vi "controlZLockIn.vi"(4 "thrAng":dbl=4.0 format="%#_13g", 6 "stop":bool, 7 "thr":dbl, 8 "error in (no error)":errorcluster, 9 "Tipo":enum16{"Amplitud", "Fase"}(ring), 10 "name":string, 11 "Distancia de medicion":dbl) -> (0 "error out":errorcluster, 1 "Act. Z":bool, 2 "limite":bool, 5 "Distancia Nano Z Act.":dbl)   [LabVIEW 2018]
uses:
  <vilib>/Utility/file.llb/Write Delimited Spreadsheet (DBL).vi
panel:
  out "Cerca":bool
  out "Fase":dbl[](graph)
  out "Thr":bool
  out "Amplitud":dbl[](graph)
  in  "stop 2":bool
  out "CambioZ":dbl
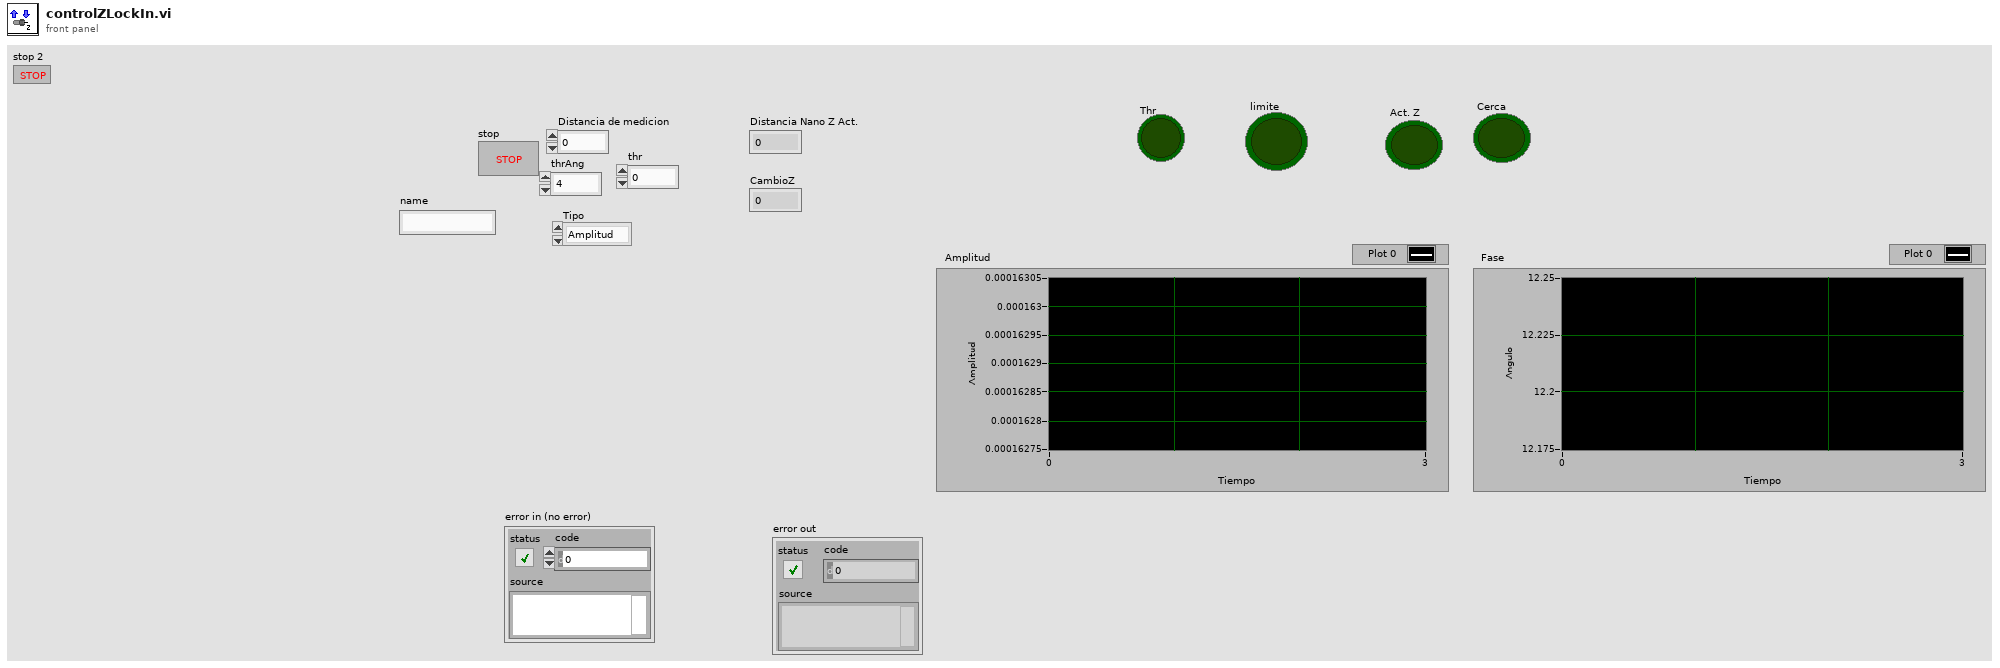
[diagram p1: front panel]
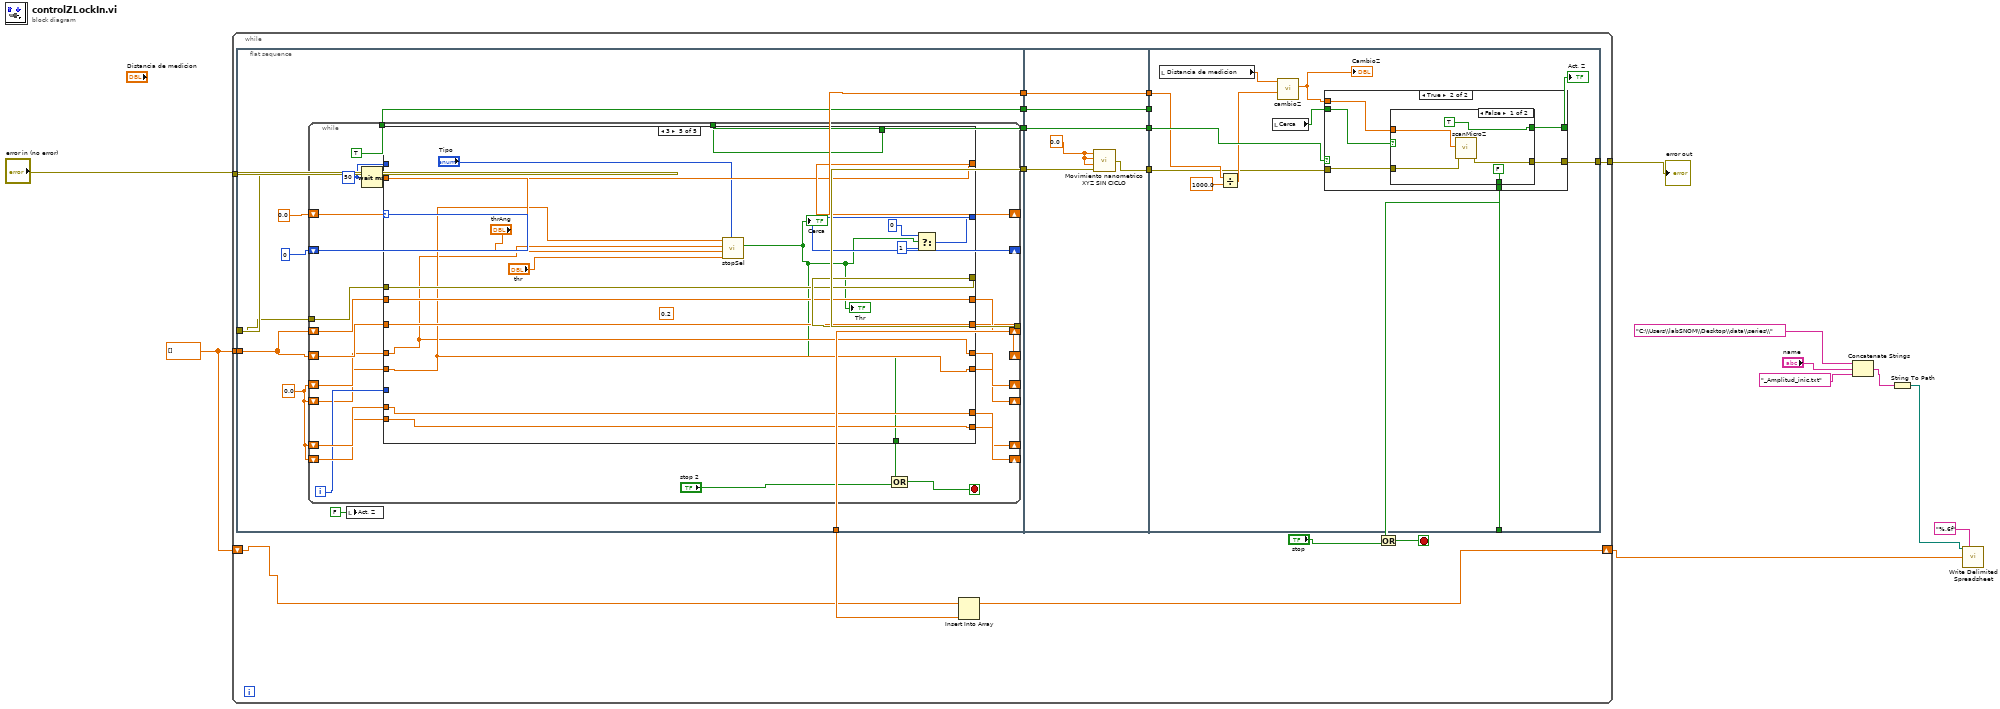
[diagram p0: block diagram]
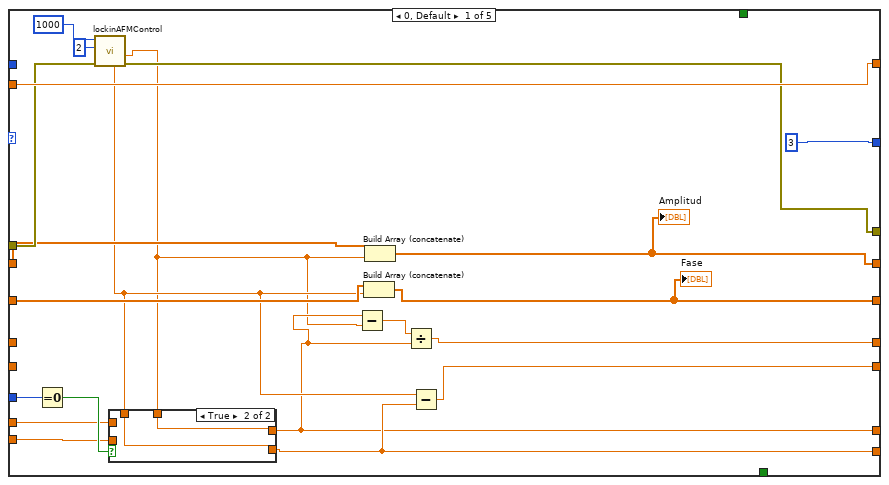
[diagram p2: hidden frame]
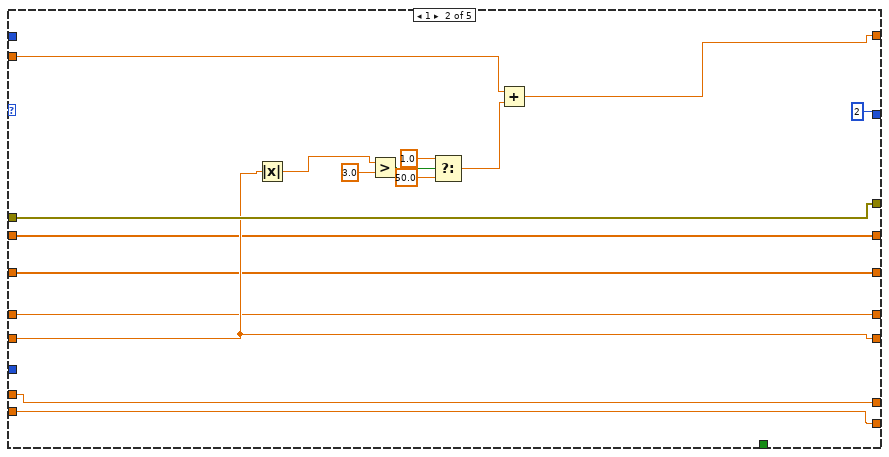
[diagram p4: hidden frame]
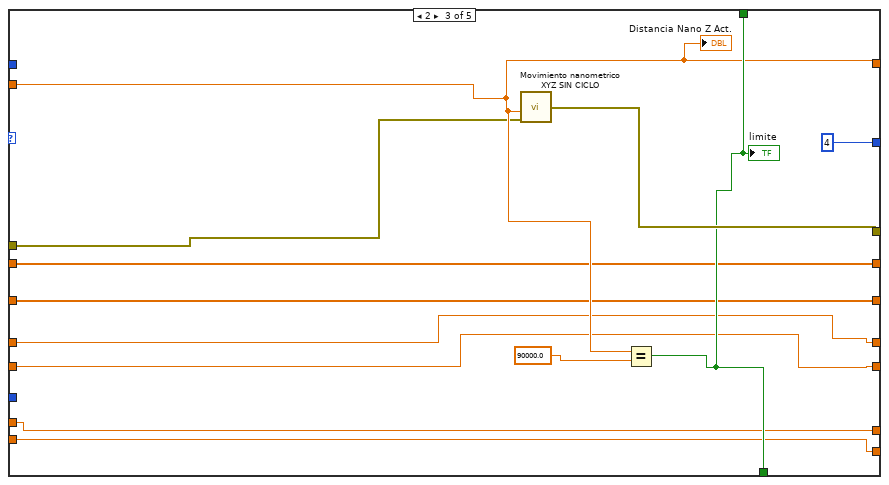
[diagram p5: hidden frame]
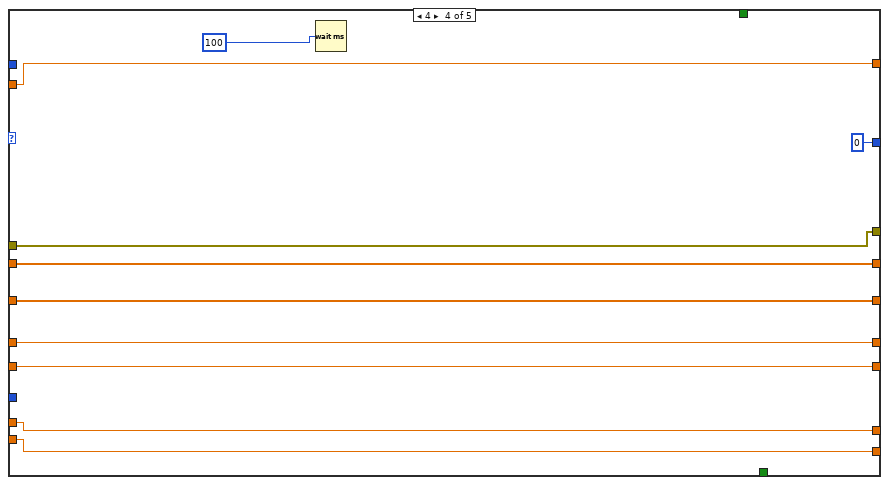
[diagram p6: hidden frame]
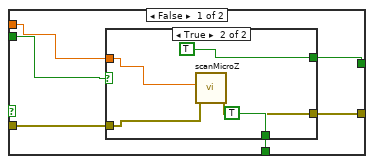
[diagram p7: hidden frame]
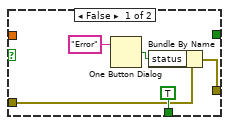
[diagram p8: hidden frame]
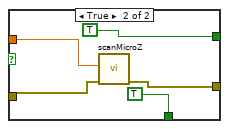
[diagram p9: hidden frame]
diagram:
  w8 = dbl[] []
  n1 = while {
    tunnel: "error in (no error)" -> [w27]
    tunnel: [w18] -> w9
    tunnel: w8 -> [w14]
    shift-right: [w11] -> w1
    shift-left: w8 -> [w12]
    stop <- w22 stop-if-true
    n2 = flat-sequence {
      tunnel: w27 -> [w30]
      tunnel: [w34] -> w24
      tunnel: [w35] -> w17
      tunnel: [w33] -> w16
      tunnel: [w32] -> w15
      tunnel: w14 -> [w29]
      tunnel: [w31] -> w13
      tunnel: [w147] -> w26
      tunnel: [w146] -> w25
      tunnel: w24 -> [w145]
      tunnel: [w145] -> w23
      tunnel: [w143] -> w19
      tunnel: w17 -> [w142]
      tunnel: w16 -> [w146]
      tunnel: w15 -> [w147]
      tunnel: w26 -> [w157]
      tunnel: w25 -> [_]
      tunnel: w23 -> [w156]
      tunnel: [w153] -> w21
      tunnel: w19 -> [w152]
      tunnel: [w151] -> w18
      frame #0 {
        w28 = 0.0
        n3 = while {
          shift-right: [w60] -> _
          shift-left: 0 -> [w63]
          shift-right: [w61] -> w34
          shift-left: 0.0 -> [w62]
          tunnel: [w59] -> w35
          tunnel: [TRUE] -> w33
          tunnel: [w55] -> w32
          shift-right: [w50] -> w31
          shift-left: w29 -> [w51]
          shift-right: [w43] -> _
          shift-left: w28 -> [w47]
          tunnel: w30 -> [w52]
          shift-right: [w48] -> _
          shift-left: w29 -> [w49]
          shift-right: [w44] -> _
          shift-left: w28 -> [w46]
          shift-right: [w42] -> _
          shift-left: w28 -> [w40]
          shift-right: [w41] -> _
          shift-left: w28 -> [w39]
          i -> [w45]
          stop <- w54 stop-if-true
          w58 = u32 50 ("milliseconds to wait")
          n4 = Wait (ms)(milliseconds to wait=w58) -> ()  [unwired: 1 out]
          n5 = case shown="3" w63 {
            tunnel: w62 -> [w84 w92 w112 w125 w140]
            tunnel: [w84 w91 w112 w125 w140] -> w61
            tunnel: w52 -> [w83 w103 w111 w123 w141]
            tunnel: [3 2 4 0 ("f") w137] -> w60
            tunnel: [w82 w103 w115 w123 w141] -> w59
            tunnel: w58 -> [_ _ _ _ _]
            tunnel: [_ _ w113 _ w127] -> w57
            tunnel: [_ _ w113 _ _] -> w55
            tunnel: w51 -> [w78 w94 w110 w122 w136]
            tunnel: [w77 w94 w110 w122 w136] -> w50
            tunnel: w49 -> [w76 w95 w109 w121 w135]
            tunnel: [w75 w95 w109 w121 w135] -> w48
            tunnel: w47 -> [w72 w90 w106 w118 w134]
            tunnel: w46 -> [w71 w89 w105 w117 w133]
            tunnel: w45 -> [w73 _ _ _ _]
            tunnel: [w68 w89 w105 w117 w133] -> w44
            tunnel: [w66 w90 w106 w118 w134] -> w43
            tunnel: [w70 w96 w108 w120 w130] -> w42
            tunnel: [w67 w97 w107 w119 w132] -> w41
            tunnel: w40 -> [_ w96 w108 w120 w130]
            tunnel: w39 -> [_ w97 w107 w119 w132]
            frame 0, Default {
              n6 = Equal To 0?(x=w73) -> (x = 0?=w74:bool)
              n7 = call "lockinAFMControl.vi"("error in"=w83, "NUMERO DE MED."=2, "milliseconds to wait"=u32 1000) -> ("error out"=w82:errorcluster, "Prom. X"=w65:dbl, "Prom. Y"=w69:dbl)  [unwired: 4 in, 2 out]
              n8 = case shown="True" w74 {
                tunnel: w72 -> [w86 _]
                tunnel: w71 -> [w85 _]
                tunnel: w69 -> [_ w88]
                tunnel: [w85 w88] -> w68
                tunnel: [w86 w87] -> w66
                tunnel: w65 -> [_ w87]
                frame False {
                }
                frame True {
                }
              }
              n9 = Subtract(x=w66, y=w65) -> (x-y=w64:dbl)
              n10 = Build Array (concatenate)(w76, w69) -> (w75:dbl[])
              "Fase" <- w75
              n11 = Build Array (concatenate)(w78, w65) -> (w77:dbl[])
              "Amplitud" <- w77
              n12 = Divide(x=w64, y=w66) -> (x/y=w70:dbl)
              n13 = Subtract(x=w69, y=w68) -> (x-y=w67:dbl)
            }
            frame 1 {
              n14 = Absolute Value(x=w97) -> (abs(x)=w98:dbl)
              n15 = Greater?(x=w98, y=3.0) -> (0:w101:bool)
              n16 = Select(t=1.0, s=w101, f=50.0) -> (s? t:f=w93:dbl)
              n17 = Add(x=w92, y=w93) -> (x+y=w91:dbl)
            }
            frame 2 {
              n18 = call "Movimiento nanometrico XYZ SIN CICLO.vi"("Error In"=w111, "Movimiento en Z"=w112) -> ("Error Out"=w115:errorcluster)  [unwired: 4 in]
              n19 = Equal?(x=w112, y=90000.0) -> (x = y?=w113:bool)
              "limite" <- w113
              "Distancia Nano Z Act." <- w112
            }
            frame 4 {
              n20 = Wait (ms)(milliseconds to wait=i64 100) -> ()  [unwired: 1 out]
            }
            frame 3 {
              (unwired) 0.2 ("y")
              n21 = call "stopSel.vi"("Tipo"="Tipo", "thr"="thr", "thr. Ang"="thrAng", "Err.Amp"=w130, "DifFase"=w132) -> ("stop"=w127:bool)  [unwired: 6 in]
              "Cerca" <- w127
              "Thr" <- w127
              n22 = Select(t=0, s=w127, f=1) -> (s? t:f=w137:i32)
            }
          }
          n23 = Compound Arithmetic op=OR(w57, "stop 2") -> (w54:bool)
        }
        n24 = local write "Act. Z"(FALSE ("Act. Z")) -> ()
      }
      frame #1 {
        w144 = 0.0
        n25 = call "Movimiento nanometrico XYZ SIN CICLO.vi"("Error In"=w142, "Movimiento en Z"=w144, "Movimiento en Y"=w144, "Movimiento en X"=w144) -> ("Error Out"=w143:errorcluster)  [unwired: 2 in]
      }
      frame #2 {
        n26 = local read "Distancia de medicion"() -> (w155:dbl)
        n27 = Divide(x=w156, y=1000.0) -> (x/y=w154:dbl)
        n28 = local read "Cerca"() -> (w148:bool)
        n29 = call "cambioZ.vi"("DISTANCIA"=w154, "TARGET"=w155) -> ("CAMBIO Z"=w149:dbl)  [unwired: 9 in]
        "CambioZ" <- w149
        n30 = case shown="True" w157 {
          tunnel: w148 -> [w162 w180]
          tunnel: w149 -> [w163 w179]
          tunnel: [w164 w178] -> w153
          tunnel: w152 -> [w161 w176]
          tunnel: [w160 w177] -> w151
          tunnel: [w159 w175] -> w150
          frame False {
            n31 = case shown="True" w162 {
              tunnel: w163 -> [_ w170]
              tunnel: [TRUE TRUE] -> w164
              tunnel: w161 -> [w167 w173]
              tunnel: [w165 w172] -> w160
              tunnel: [_ TRUE ("Activar movimiento en Z")] -> w159
              frame False {
                n32 = One Button Dialog(message="Error") -> (true=w166:bool)  [unwired: 1 in]
                n33 = Bundle By Name(cluster=w167, "status"=w166) -> (w165:errorcluster)
              }
              frame True {
                n34 = call "scanMicroZ.vi"("error in (no error)"=w173, "Mov Z"=w170) -> ("error out"=w172:errorcluster)  [unwired: 9 in]
              }
            }
          }
          frame True {
            n35 = case shown="False" w180 {
              tunnel: w179 -> [w181 w190]
              tunnel: [FALSE TRUE] -> w178
              tunnel: [w184 w188] -> w177
              tunnel: w176 -> [w183 w187]
              tunnel: [TRUE ("Activar movimiento en Z") TRUE ("Activar movimiento en Z")] -> w175
              frame False {
                n36 = call "scanMicroZ.vi"("error in (no error)"=w183, "Mov Z"=w181) -> ("error out"=w184:errorcluster)  [unwired: 9 in]
              }
              frame True {
                n37 = call "scanMicroZ.vi"("error in (no error)"=w187, "Mov Z"=w190) -> ("error out"=w188:errorcluster)  [unwired: 9 in]
              }
            }
          }
        }
        "Act. Z" <- w150
      }
    }
    n38 = Insert Into Array(array=w12, new element=w13) -> (w11:dbl[])  [unwired: 1 in]
    n39 = Or(x=w21, y="stop") -> (x .or. y?=w22:bool)
  }
  "error out" <- w9
  n40 = Concatenate Strings("C:\\Users\\labSNOM\\Desktop\\data\\series\\", "name", "_Amplitud_inic.txt") -> (w3:string)
  n41 = String To Path(string=w3) -> (path=w2:path)
  n42 = call-poly <vilib>:"Write Delimited Spreadsheet.vi"("file path (dialog if empty)"=w2, "format (%.3f)"="%.6f", "1D data"=w1) -> ()  [unwired: 11 in, 2 out]
